vi "Pre Launch Init.vi"(11 "Sequencer in":refnum<class "Sequencer.lvclass">) -> (0 "error out":errorcluster, 3 "Sequencer out":refnum<class "Sequencer.lvclass">)   [LabVIEW 2015, in "Sequencer.lvlib" / "Sequencer.lvclass"]
doc: "(<B>Filename</B>: Actor Framework.lvlib:Actor.lvclass:Pre Launch Init.vi)\n\nDefines behavior that occurs after the Launch Nested Actor method is invoked but before the actor's Actor Core method begins running.\n\nBy default, this method does nothing. A descendant class may override it to define behavior."
uses:
  Sequencer.lvclass
  <userlib>/_Win8uiFramework/ViewableActor.lvclass
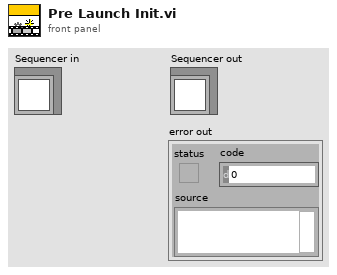
[diagram p1: front panel]
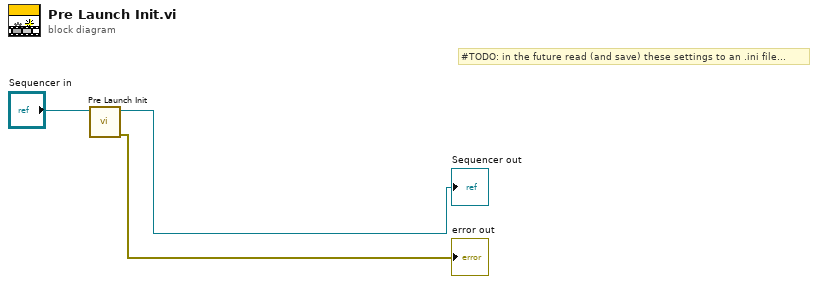
[diagram p0: block diagram]
diagram:
  # "#TODO: in the future read (and save) these settings to an .ini file..."
  n1 = call-parent "Pre Launch Init.vi"("ViewableActor in"="Sequencer in") -> ("error out"=→"error out":errorcluster, "ViewableActor out"=→"Sequencer out":refnum<class "Sequencer.lvclass">)  [unwired: 9 in]
